vi "Semaphore Release Destroy.vi"(8 "error in":errorcluster, 11 "TDM IO Lock":u16) -> (0 "error out":errorcluster)   [LabVIEW 2011]
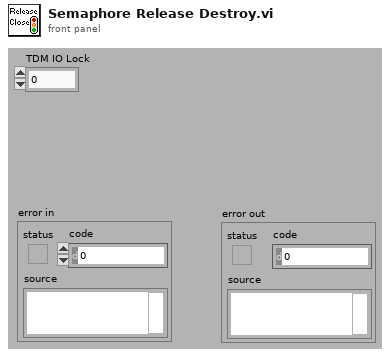
[diagram p1: front panel]
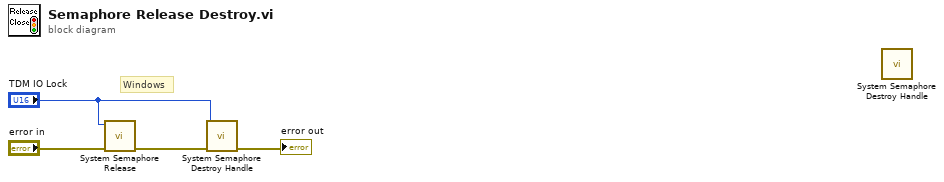
[diagram p0: block diagram]
diagram:
  # "Windows"
  n1 = call "System Semaphore Release.vi"("error in (no error)"="error in", "SemaphoreHandle"="TDM IO Lock") -> ("error out"=w1:errorcluster)  [unwired: 8 in, 1 out]
  n2 = call "System Semaphore Destroy Handle.vi"("error in (no error)"=w1, "SemaphoreHandle"="TDM IO Lock") -> ("error out"=→"error out":errorcluster)  [unwired: 9 in]
  n3 = call "System Semaphore Destroy Handle.vi"() -> ()  [unwired: 11 in, 1 out]
